vi "PeriodicFilter-Filtered Entry.vi"(11 "Data In":T1 {"LastCheckT" format="%<%.3X>T"}) -> (2 "Entry":T2[](array[typedef]), 3 "Data Out":T1 {"LastCheckT" format="%<%.3X>T"})   [LabVIEW 2017, in "Communicable State Machine.lvlib"]
uses:
  Communicable State Machine.lvlib
  Periodic String Filter Info.ctl
  Periodic String Filter Data.ctl
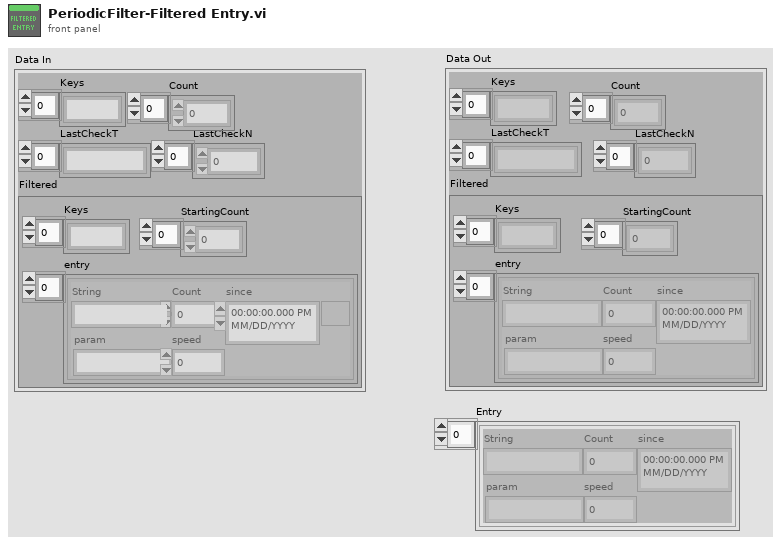
[diagram p1: front panel]
types:
  T1 = typedef "Communicable State Machine.lvlib/Periodic String Filter Data.ctl" = cluster{"Keys":string[], "Count":i64[], "LastCheckT":timestamp[], "LastCheckN":i64[], "Filtered":cluster{"Keys":string[], "StartingCount":i64[], "entry":T2[]}}
  T2 = typedef "Communicable State Machine.lvlib/Periodic String Filter Info.ctl" = cluster{"String":string, "Count":i64, "since":timestamp, "param":string, "speed":dbl}
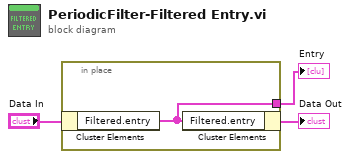
[diagram p0: block diagram]
diagram:
  n1 = in-place {
    in-place-border: [w4] -> w3
    n2 = in-place-cluster #1("Data In") -> ("Filtered.entry"=w4:T2[])
    n3 = in-place-cluster #1("Filtered.entry"=w4) -> (→"Data Out":T1)
  }
  "Entry" <- w3
